vi "Project - Name.vi"(7 "Msg Chain":string, 8 "error in (no error)":errorcluster {"code" format="Error %.0f"}, 10 "Project Doc":refnum<class "Project Documentation.lvclass">, 11 "VIDoc Printer - Confluence In":refnum<class "VIDoc Printer - Confluence.lvclass">) -> (0 "error out":errorcluster {"code" format="Error %.0f"}, 3 "VIDoc Printer - Confluence Out":refnum<class "VIDoc Printer - Confluence.lvclass">)   [LabVIEW 2023, in "VIDoc Printer - Confluence.lvlib" / "VIDoc Printer - Confluence.lvclass"]
uses:
  VIDoc Printer - Confluence.lvclass
  C:/projects/DMC/Tooling/Git-Action-Service/Source/Documentation Generation/Printers/Printer/VIDoc Printer.lvclass
  Parsing/Project Documentation/Project Documentation.lvclass
  Confluence Formatting/Types/Format Combo Box.ctl
  Parsing/Project Documentation/Project Documentation.lvclass/Project Documentation.ctl
  Printer/VIDoc Printer.lvclass/VIDoc Printer.ctl
  VIDoc Printer - Confluence.lvclass/VIDoc Printer - Confluence.ctl
  Printer/Accessors/Get Project Settings - Paths.vi
  Accessors/Get Working Directory.vi
  Parsing/Project Documentation/Get Name.vi
  Parsing/Project Documentation/Get Path.vi
  Confluence Formatting/Confluence Formatting.lvlib
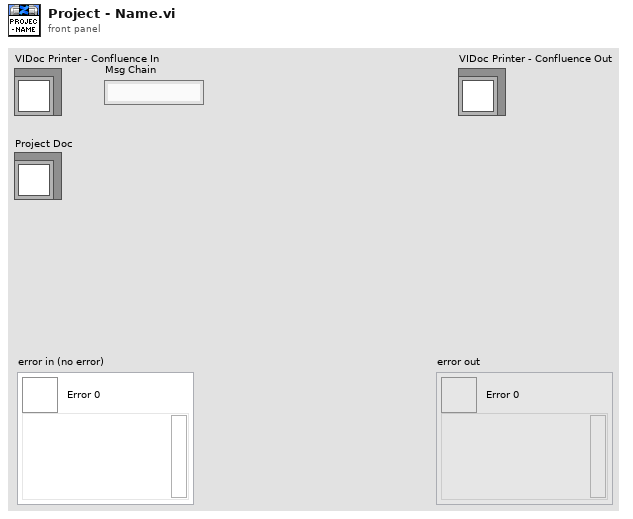
[diagram p1: front panel]
types:
  T1 = typedef "Confluence Formatting.lvlib/Format Combo Box.ctl" = string
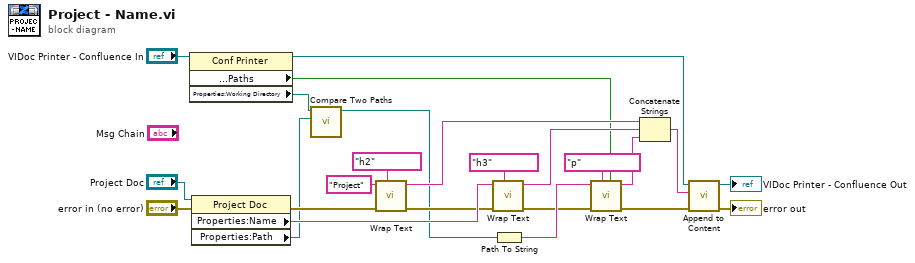
[diagram p0: block diagram]
diagram:
  n1 = property class="Conf Printer"(reference="VIDoc Printer - Confluence In") -> (reference out=w15:refnum<class "VIDoc Printer - Confluence.lvclass">, "Properties:Settings:Projects:Paths"=w4:bool, "Properties:Working Directory"=w3:path)  [unwired: 1 in, 1 out]
  n2 = property class="Project Doc"(reference="Project Doc", error in="error in (no error)") -> (error out=w18:errorcluster, "Properties:Name"=w20:string, "Properties:Path"=w2:path)  [unwired: 1 out]
  n3 = call <vilib>:"Compare Two Paths.vi"("Path 2"=w2, "Path 1"=w3) -> ("Relative Path from 1 to 2"=w1:path)  [unwired: 6 in, 3 out]
  n4 = call "Wrap Text.vi"("Formatting"=T1 "h2", "Error in"=w18, "String"="Project") -> ("Error out"=w13:errorcluster, "Wrapped String"=w17:string)  [unwired: 7 in]
  n5 = call "Wrap Text.vi"("Formatting"=T1 "h3", "Error in"=w13, "String"=w20) -> ("Error out"=w12:errorcluster, "Wrapped String"=w16:string)  [unwired: 7 in]
  n6 = Path To String(path=w1) -> (string=w14:string)
  n7 = call "Wrap Text.vi"("Enabled? (T)"=w4, "Formatting"=T1 "p", "Error in"=w12, "String"=w14) -> ("Error out"=w10:errorcluster, "Wrapped String"=w11:string)  [unwired: 6 in]
  n8 = Concatenate Strings(w17, w16, w11) -> (w9:string)
  n9 = call "Append to Content.vi"("error in (no error)"=w10, "Content"=w9, "VIDoc Printer - Confluence In"=w15) -> ("error out"=→"error out":errorcluster, "VIDoc Printer - Confluence Out"=→"VIDoc Printer - Confluence Out":refnum<class "VIDoc Printer - Confluence.lvclass">)  [unwired: 7 in]
